vi "Limit_Safety.vi"(1 "Disable_Limit_Safeties":bool, 3 "Outer_Arm_Pivot_Throttle":dbl, 4 "Lower_Limit":dbl, 5 "Upper_Limit":dbl, 6 "Sensor_Value":dbl) -> (0 "Corrected Output":dbl)   [LabVIEW 2020]
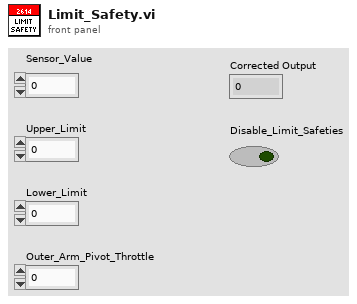
[diagram p1: front panel]
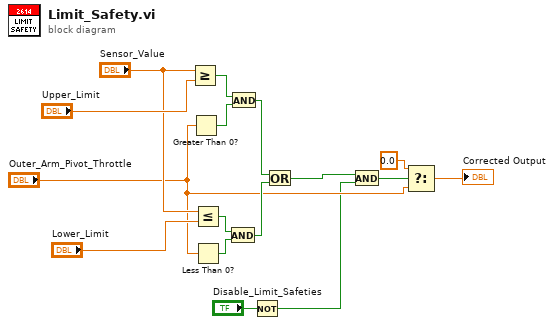
[diagram p0: block diagram]
diagram:
  n1 = Greater Or Equal?(x="Sensor_Value", y="Upper_Limit") -> (x >= y?=w15:bool)
  n2 = Greater Than 0?(x="Outer_Arm_Pivot_Throttle") -> (x > 0?=w14:bool)
  n3 = Less Or Equal?(x="Sensor_Value", y="Lower_Limit") -> (x <= y?=w11:bool)
  n4 = Less Than 0?(x="Outer_Arm_Pivot_Throttle") -> (x < 0?=w10:bool)
  n5 = And(x=w11, y=w10) -> (x .and. y?=w8:bool)
  n6 = And(x=w15, y=w14) -> (x .and. y?=w9:bool)
  n7 = Not(x="Disable_Limit_Safeties") -> (.not. x?=w1:bool)
  n8 = Or(x=w9, y=w8) -> (x .or. y?=w7:bool)
  n9 = And(x=w7, y=w1) -> (x .and. y?=w3:bool)
  n10 = Select(t=0.0, s=w3, f="Outer_Arm_Pivot_Throttle") -> (s? t:f=→"Corrected Output":dbl)
